vi "Define 2D Heat PDE Domain (Rect).vi"(0 "PDE in":refnum<class "NI_PDE.lvclass">, 5 "T":T3={"initial t"=0.0, "final t"=1.0, "# of t-points"=11}, 7 "X":T2={"start x"=0.0, "end x"=1.0, "# of x-points"=11}, 9 "Y":T1={"start y"=0.0, "end y"=1.0, "# of y-points"=11}, 11 "error in (no error)":errorcluster) -> (4 "PDE out":refnum<class "NI_PDE.lvclass">, 15 "error out":errorcluster)   [LabVIEW 2017, in "NI_PDE.lvlib"]
doc: "Defines the domain where you solve the partial differential equation. You must manually select the polymorphic instance to use."
uses:
  <vilib>/gmath/NI_PDE.lvlib
  <vilib>/gmath/pde.llb/PDEClass/NI_PDE.lvclass
  <vilib>/gmath/pde.llb/PDEClass/PDE_Heat_2D/NI_PDE_Heat_2D.lvclass
  e:/builds/penguin/labview/branches/2017/dev/dist/vi.lib/gmath/pde.llb/PDEClass/NI_PDE.lvclass
  <vilib>/gmath/pde.llb/DomainClass/Domain_Evolut_2D_Rect/NI_Domain_Evolut_2D_Rect.lvclass
  e:/builds/penguin/labview/branches/2017/dev/dist/vi.lib/gmath/pde.llb/DomainClass/NI_Domain.lvclass
  <vilib>/gmath/pde.llb/DomainClass/Domain_Evolut_2D_Rect/Domain Data.ctl
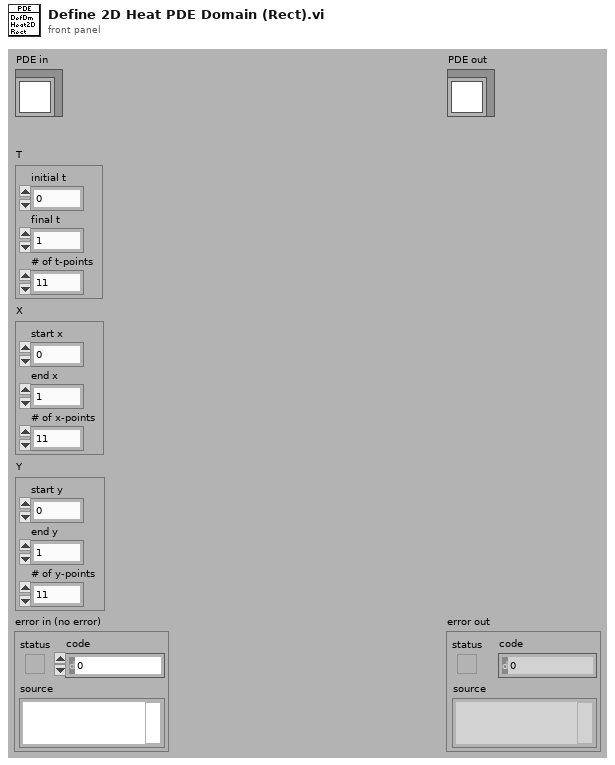
[diagram p1: front panel]
types:
  T1 = cluster{"start y":dbl, "end y":dbl, "# of y-points":i32}
  T2 = cluster{"start x":dbl, "end x":dbl, "# of x-points":i32}
  T3 = cluster{"initial t":dbl, "final t":dbl, "# of t-points":i32}
  T4 = typedef "NI_PDE.lvlib/NI_Domain_Evolut_2D_Rect.lvclass/Domain Data.ctl" = cluster{"T":cluster{"initial t":dbl, "final t":dbl, "# of t-points":i32}, "X":cluster{"start x":dbl, "end x":dbl, "# of x-points":i32}, "Y":cluster{"start y":dbl, "end y":dbl, "# of y-points":i32}}
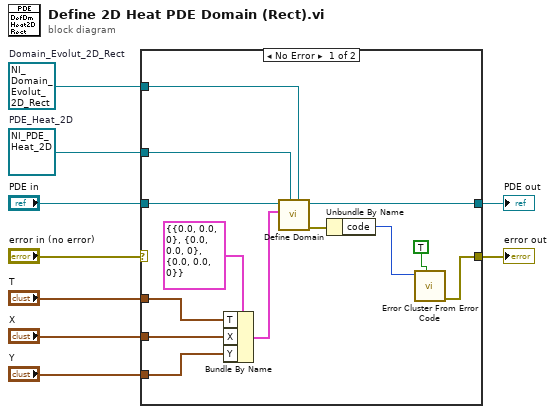
[diagram p0: block diagram]
diagram:
  w1 = refnum<class "NI_Domain_Evolut_2D_Rect.lvclass"> refnum  # Domain_Evolut_2D_Rect
  w2 = refnum<class "NI_PDE_Heat_2D.lvclass"> refnum  # PDE_Heat_2D
  n1 = case shown="No Error" "error in (no error)" {
    selector: "error in (no error)" -> [_ w24]
    tunnel: "PDE in" -> [w17 w23]
    tunnel: [w19 w23] -> w8
    tunnel: "Y" -> [w11 _]
    tunnel: "X" -> [w12 _]
    tunnel: "T" -> [w13 _]
    tunnel: [w20 w24] -> w4
    tunnel: w2 -> [w16 _]
    tunnel: w1 -> [w15 _]
    frame No Error {
      n2 = Bundle By Name(cluster=T4 {"T"={"initial t"=0.0, "final t"=0.0, "# of t-points"=0}, "X"={"start x"=0.0, "end x"=0.0, "# of x-points"=0}, "Y"={"start y"=0.0, "end y"=0.0, "# of y-points"=0}} ("domain data"), "T"=w13, "X"=w12, "Y"=w11) -> (w10:T4)
      n3 = call <vilib>:"Define Domain.vi"("target Domain"=w15, "target PDE"=w16, "domain"=w10, "PDE in"=w17) -> ("error out"=w18:errorcluster, "PDE out"=w19:refnum<class "NI_PDE.lvclass">)  [unwired: 1 in, 5 out]
      n4 = Unbundle By Name(w18) -> ("code"=w22:i32)
      n5 = call <vilib>:"Error Cluster From Error Code.vi"("show call chain? (False)"=TRUE, "error code (0)"=w22) -> ("error out"=w20:errorcluster)  [unwired: 1 in, 6 out]
    }
    frame Error {
    }
  }
  "PDE out" <- w8
  "error out" <- w4
